vi "Passing Parameters Integer.vi"(10 "y":i32, 11 "x":i32) -> (3 "function return":i32)   [LabVIEW 2018, in "ParsingDataSampleDLL.lvlib"]
doc: "__declspec(dllexport) int PassingParameters_Integer (int x, int y);"
uses:
  ParsingDataSampleDLL.lvlib
  ni_reference_vs/Debug/ParsingDataSampleDLL.dll
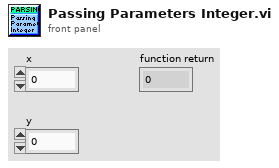
[diagram p1: front panel]
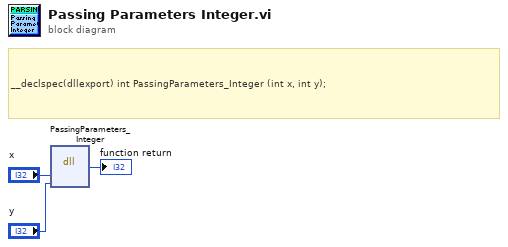
[diagram p0: block diagram]
diagram:
  # "__declspec(dllexport) int PassingParameters_Integer (int x, int y);"
  n1 = dll-call lib="C:/Users/celit/Documents/GitHub/Labview_Python_DLL_Call/ni_reference_vs/Debug/ParsingDataSampleDLL.*" fn="PassingParameters_Integer"("x"="x", "y"="y") -> (→"function return":i32)  [unwired: 5 in, 2 out]
